vi "OE2031&OE2041_RS232_Query Data.vi"(0 "VISA resource name":refnum<visa-resource-name>, 11 "Error in (no error)":errorcluster caption="error out（no error）") -> (4 "VISA resource  out":refnum<visa-resource-name>, 6 "Data Array":dbl[](array[numeric]), 8 "Parameter Values":T1, 10 "Output String":string, 15 "Error out":errorcluster caption="error out")   [LabVIEW 2011]
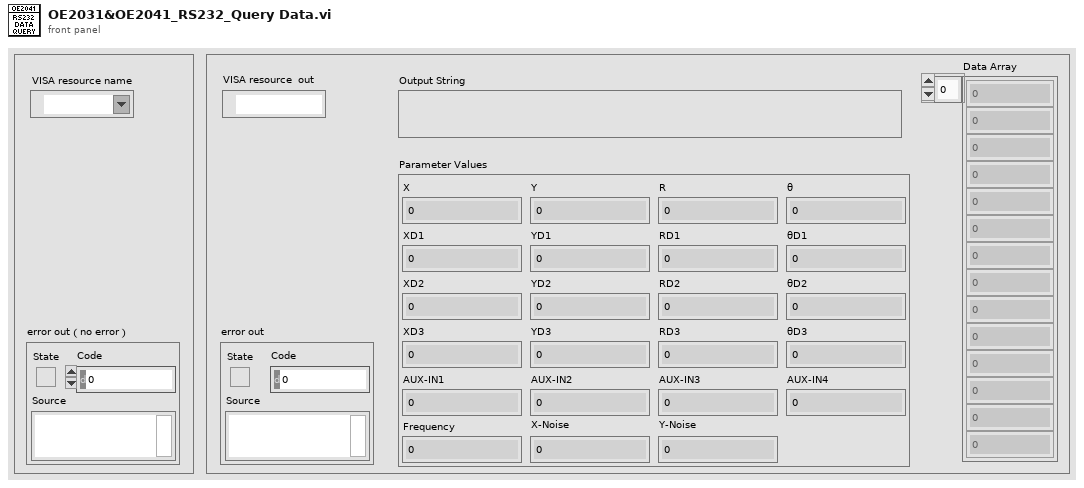
[diagram p1: front panel]
types:
  T1 = cluster{"X":dbl, "Y":dbl, "R":dbl, "θ":dbl, "Frequency":dbl, "XD1":dbl, "YD1":dbl, "RD1":dbl, "θD1":dbl, "XD2":dbl, "YD2":dbl, "RD2":dbl, "θD2":dbl, "XD3":dbl, "YD3":dbl, "RD3":dbl, "θD3":dbl, "X-Noise":dbl, "Y-Noise":dbl, "AUX-IN1":dbl, "AUX-IN2":dbl, "AUX-IN3":dbl, "AUX-IN4":dbl}
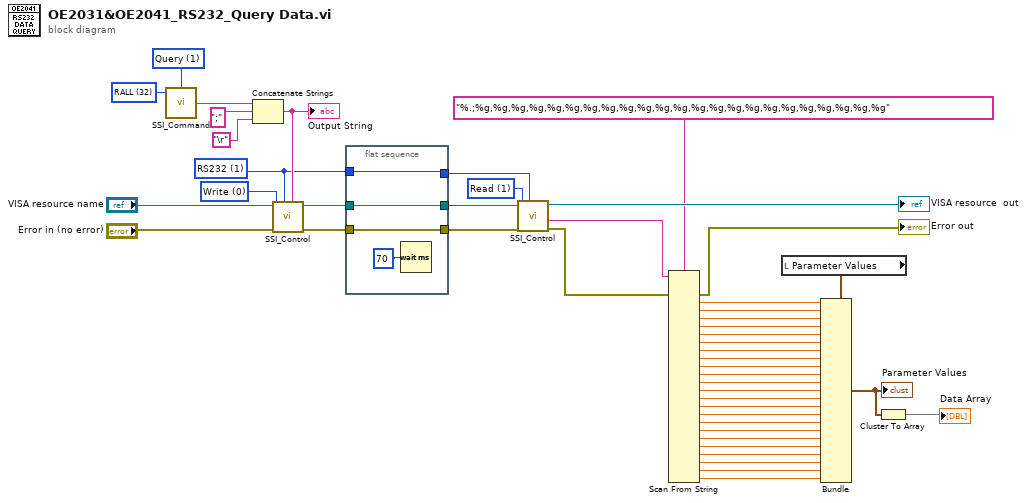
[diagram p0: block diagram]
diagram:
  w6 = u16 1 items=["USB"=0, "RS232"=1, "Ethernet"=3] ("Remote Mode")
  w8 = u16 32 items=["ISRC", "IGND", "ICPL", "ILIN", "PHAS", "FMOD", "RSLP", "FREQ", "SWPT", "SLLM", "SULM", "SSLL", "SSLG", "STLM", "SWRM", "IRNG", "SENS", "RMOD", "OFLT", "OFSL", "SYNC", "DMOD", "HARM", "DARB", "SWVT", "SLVL", "SVLL", "SVUL", "SVSL", "SVSG", "SVTM", "SVRM", "RALL", "SNAP", "OUTP", "OAUX", "COUT", "CAUX", "COFP", "CEXP", "FPOP", "OEXP", "*IDN", "*RST", "OVLD", "INOV", "GNOV", "*PLL", "SSET", "RSET", "AGAN", "APHS", "ARSV", "ASCL", "EQCD", "EQCS", "SPED", "SRAT", "SLEN", "SSLE", "STRG", "SPRM", "STRD", "PAUS", "RSET", "SPTS", "TRCA", "TEMP", "RSTU", "INHZ", "DEQU", "SADD", "ARNG", "CSPE", "ISRCD", "IGNDD", "ICPLD", "ILIND", "PHASD", "FMODD", "RSLPD", "FREQD", "SWPTD", "SLLMD", "SULMD", "SSLLD", "SSLGD", "STLMD", "SWRMD", "SENSD", "RMODD", "OFLTD", "OFSLD", "SYNCD", "HARMD", "EQCDD", "EQCSD", "SNAPD", "OUTPD", "SWVTD", "SLVLD", "SVLLD", "SVULD", "SVSLD", "SVSGD", "SVTMD", "SVRMD", "SVDCD", "ARSVD", "AGAND", "APHSD", "ASCLD", "FPOPD", "CAUXD", "OEXPD", "SPEDD", "SRATD", "SLEND", "SSLED", "STRGD", "SPRMD", "STRDD", "PAUSD", "RESTD", "SPTSD", "TRCAD", "*IDND", "*RSTD", "INOVD", "GNOVD", "*PLLD", "SSETD", "RSETD", "RALLD"] ("Command Type")
  w4 = u16 1 items=["Set", "Query"] ("Opera")
  w39 = u16 1 items=["Write", "Read"] ("Control")
  w44 = u16 0 items=["Write", "Read"] ("Control")
  n1 = call "SSI_Command.vi"("Opera"=w4, "Command Type"=w8) -> ("Output string"=w7:string)  [unwired: 2 in]
  n2 = Concatenate Strings(w7, ";" ("字符串"), "\r") -> (w10:string)
  "Output String" <- w10
  n3 = call "SSI_Control.vi"("Write Buffer"=w10, "Remote Mode"=w6, "Error in (no error)"="Error in (no error)", "Control"=w44, "VISA resource name"="VISA resource name") -> ("Error out"=w42:errorcluster, "VISA resource  out"=w43:refnum<visa-resource-name>)  [unwired: 3 in, 2 out]
  n4 = flat-sequence {
    tunnel: w43 -> [w51]
    tunnel: w42 -> [w50]
    tunnel: [w51] -> w41
    tunnel: [w50] -> w40
    tunnel: [w48] -> w38
    tunnel: w6 -> [w48]
    frame #0 {
      n5 = Wait (ms)(milliseconds to wait=u32 70 ("等待时间（毫秒）")) -> ()  [unwired: 1 out]
    }
  }
  n6 = call "SSI_Control.vi"("Remote Mode"=w38, "Error in (no error)"=w40, "Control"=w39, "VISA resource name"=w41) -> ("Error out"=w37:errorcluster, "Read Buffer"=w5:string, "VISA resource  out"=→"VISA resource  out":refnum<visa-resource-name>)  [unwired: 4 in, 1 out]
  n7 = Scan From String(format string="%.;%g,%g,%g,%g,%g,%g,%g,%g,%g,%g,%g,%g,%g,%g,%g,%g,%g,%g,%g,%g,%g,%g,%g" ("格式字符串"), input string=w5, error in=w37) -> (error out=→"Error out":errorcluster, output 1=w35:dbl, output 2=w34:dbl, output 3=w33:dbl, output 4=w32:dbl, output 5=w31:dbl, output 6=w27:dbl, output 7=w26:dbl, output 8=w25:dbl, output 9=w24:dbl, output 10=w23:dbl, output 11=w22:dbl, output 12=w18:dbl, output 13=w17:dbl, output 14=w16:dbl, output 15=w15:dbl, output 16=w14:dbl, output 17=w13:dbl, output 18=w12:dbl, output 19=w19:dbl, output 20=w20:dbl, output 21=w21:dbl, output 22=w28:dbl, output 23=w9:dbl)  [unwired: 24 in, 2 out]
  n8 = local read "Parameter Values"() -> (w29:T1)
  n9 = Bundle(cluster=w29, "X"=w35, "Y"=w34, "R"=w33, "θ"=w32, "Frequency"=w31, "XD1"=w27, "YD1"=w26, "RD1"=w25, "θD1"=w24, "XD2"=w23, "YD2"=w22, "RD2"=w18, "θD2"=w17, "XD3"=w16, "YD3"=w15, "RD3"=w14, "θD3"=w13, "X-Noise"=w12, "Y-Noise"=w19, "AUX-IN1"=w20, "AUX-IN2"=w21, "AUX-IN3"=w28, "AUX-IN4"=w9) -> (w2:T1)
  "Parameter Values" <- w2
  n10 = Cluster To Array(cluster=w2) -> (array=→"Data Array":dbl[])
